vi "updateExpMeasurementSD.vi"(3 "error in (no error)":errorcluster, 4 "Cluster control":T1, 5 "Notifier measurement":bool, 6 "Experiment in":refnum<class "Experiment.lvclass">) -> (0 "error out":errorcluster, 1 "Operate":bool, 2 "Experiment out":refnum<class "Experiment.lvclass">)   [LabVIEW 2015]
uses:
  controls/clustercontrols-measerument.ctl
  Classes/Experiment.lvclass
  globalVarSD.vi
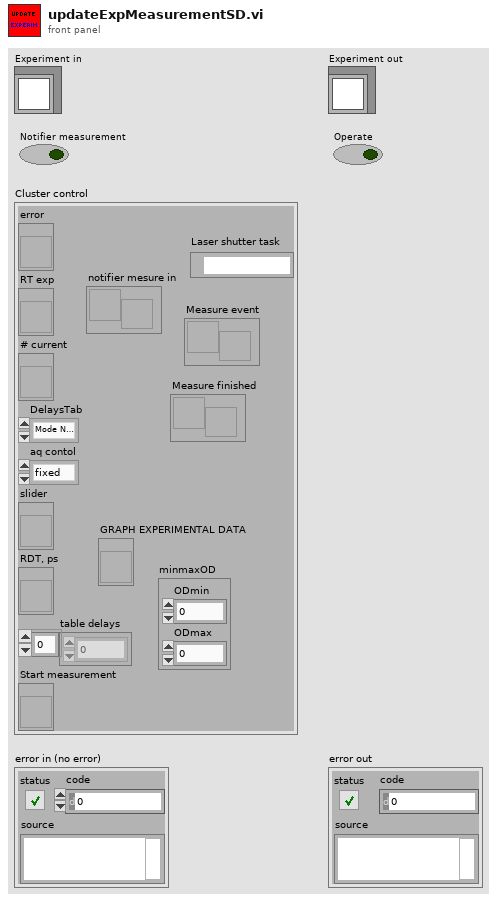
[diagram p1: front panel]
types:
  T1 = typedef "clustercontrols-measerument.ctl" = cluster{"error":refnum<vi>, "RT exp":refnum<vi>, "# current":refnum<vi>, "Start measurement":refnum<vi>, "GRAPH EXPERIMENTAL DATA":refnum<vi>, "DelaysTab":enum32{"Mode Normale", "Table"}, "slider":refnum<vi>, "aq contol":enum32{"fixed", "automatic", "fixed-auto"}, "RDT, ps":refnum<vi>, "table delays":dbl[], "notifier mesure in":refnum<notifier>, "Measure finished":refnum<user-event>, "Measure event":refnum<user-event>, "Laser shutter task":refnum<k21>, "minmaxOD":cluster{"ODmin":dbl, "ODmax":dbl}}
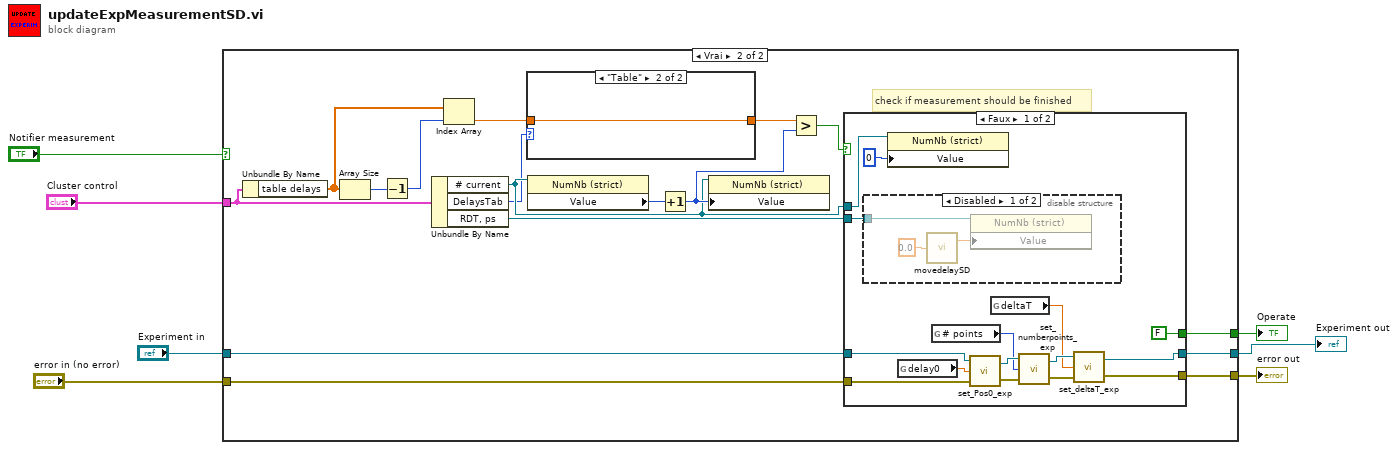
[diagram p0: block diagram]
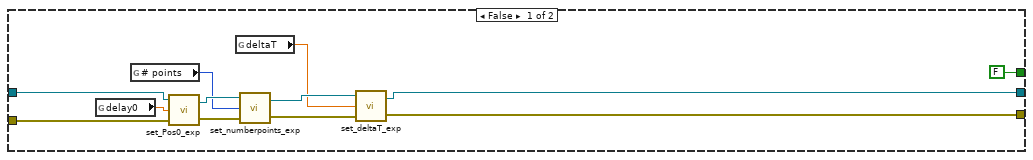
[diagram p2: hidden frame]
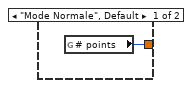
[diagram p3: hidden frame]
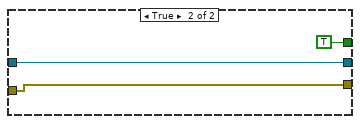
[diagram p5: hidden frame]
diagram:
  n1 = case shown="Vrai" "Notifier measurement" {
    tunnel: [FALSE ("Operate") w35] -> w3
    tunnel: "Experiment in" -> [w14 w34]
    tunnel: [w13 w32] -> w4
    tunnel: "Cluster control" -> [_ w20]
    tunnel: "error in (no error)" -> [w9 w26]
    tunnel: [w8 w25] -> w5
    frame False {
      n2 = global read "globalVarSD.vi" "delay0"() -> (w12:dbl)
      n3 = global read "globalVarSD.vi" "# points"() -> (w10:i32)
      n4 = call-dynamic "set_Pos0_exp.vi"("error in (no error)"=w9, "Pos0,ps"=w12, "Experiment.lvclass in"=w14) -> ("error out"=w16:errorcluster, "Experiment.lvclass out"=w17:refnum<class "Experiment.lvclass">)
      n5 = global read "globalVarSD.vi" "deltaT"() -> (w11:dbl)
      n6 = call-dynamic "set_numberpoints_exp.vi"("error in (no error)"=w16, "numberpoints"=w10, "Experiment.lvclass in"=w17) -> ("error out"=w15:errorcluster, "Experiment.lvclass out"=w18:refnum<class "Experiment.lvclass">)
      n7 = call-dynamic "set_deltaT_exp.vi"("error in (no error)"=w15, "deltaTlast"=w11, "Experiment.lvclass in"=w18) -> ("error out"=w8:errorcluster, "Experiment.lvclass out"=w13:refnum<class "Experiment.lvclass">)
    }
    frame True {
      # "check if measurement should be finished"
      n8 = Unbundle By Name(w20) -> ("table delays"=w22:dbl[])
      n9 = Array Size(array=w22) -> (size(s)=w24:i32)
      n10 = Decrement(x=w24) -> (x-1=w23:i32)
      n11 = Unbundle By Name(w20) -> ("# current"=w29:refnum<vi>, "DelaysTab"=w28:enum32{"Mode Normale", "Table"}, "RDT, ps"=w27:refnum<vi>)
      n12 = Index Array(array=w22, index=w23) -> (element=w21:dbl)
      n13 = case shown="\"Table\"" w28 {
        tunnel: [w37 w38] -> w31
        tunnel: w21 -> [_ w38]
        frame "Mode Normale", Default {
          n14 = global read "globalVarSD.vi" "# points"() -> (w37:i32)
        }
        frame "Table" {
        }
      }
      n15 = property class="NumNb (strict)"(reference=w29) -> ("Value"=w33:i32)  [unwired: 1 in, 2 out]
      n16 = Increment(x=w33) -> (x+1=w30:i32)
      n17 = property class="NumNb (strict)"(reference=w29, "Value"=w30) -> ()  [unwired: 1 in, 2 out]
      n18 = Greater?(x=w31, y=w30) -> (0:w36:bool)
      n19 = case shown="Faux" w36 {
        tunnel: w34 -> [w44 w58]
        tunnel: [FALSE ("Operate") TRUE ("Operate")] -> w35
        tunnel: w27 -> [w52 _]
        tunnel: w29 -> [w50 _]
        tunnel: [w41 w58] -> w32
        tunnel: w26 -> [w40 w57]
        tunnel: [w39 w57] -> w25
        frame False {
          n20 = disable-structure shown="Disabled" {
            disable-tunnel: w52 -> [w54 _]
            frame Disabled {
              n21 = call "movedelaySD.vi"("Delay, mm"=0.0) -> ("Real delay time, ps"=w56:dbl)  [unwired: 1 out]
              n22 = property class="NumNb (strict)"(reference=w54, "Value"=w56) -> ()  [unwired: 1 in, 2 out]
            }
            frame Enabled {
            }
          }
          n23 = property class="NumNb (strict)"(reference=w50, "Value"=0 ("Nombre de point indic")) -> ()  [unwired: 1 in, 2 out]
          n24 = global read "globalVarSD.vi" "delay0"() -> (w43:dbl)
          n25 = global read "globalVarSD.vi" "# points"() -> (w42:i32)
          n26 = call-dynamic "set_Pos0_exp.vi"("error in (no error)"=w40, "Pos0,ps"=w43, "Experiment.lvclass in"=w44) -> ("error out"=w47:errorcluster, "Experiment.lvclass out"=w48:refnum<class "Experiment.lvclass">)
          n27 = global read "globalVarSD.vi" "deltaT"() -> (w45:dbl)
          n28 = call-dynamic "set_numberpoints_exp.vi"("error in (no error)"=w47, "numberpoints"=w42, "Experiment.lvclass in"=w48) -> ("error out"=w46:errorcluster, "Experiment.lvclass out"=w49:refnum<class "Experiment.lvclass">)
          n29 = call-dynamic "set_deltaT_exp.vi"("error in (no error)"=w46, "deltaTlast"=w45, "Experiment.lvclass in"=w49) -> ("error out"=w39:errorcluster, "Experiment.lvclass out"=w41:refnum<class "Experiment.lvclass">)
        }
        frame True {
        }
      }
    }
  }
  "error out" <- w5
  "Experiment out" <- w4
  "Operate" <- w3
